vi "Festo.vi"(0 "CloseVi?":bool) -> ()   [LabVIEW 2011]
uses:
  GlobalVariables.vi
panel:
  in  "Valve Mode":bool
  in  "DeviceNet Reset":bool
  in  "DeviceNet HaltScanner":bool
  in  "DeviceNet DisableNetwork":bool
  in  "DeviceNet Fault":bool
  out "DnetPowerDetect":bool
  out "DupNodeFail":bool
  out "CommFailure":bool
  out "Autoverify":bool
  out "DeviceFailure":bool
  out "DisableNetwork":bool
  out "Fault":bool
  out "Run":bool
  out "FB8 Status":bool
  out "FB7 Status":bool
  out "FB6 Status":bool
  out "FB5 Status":bool
  out "FB4 Status":bool
  out "FB3 Status":bool
  out "FB2 Status":bool
  out "FB1 Status":bool
  in  "Close All Valves":bool
  in  "66":bool
  in  "68":bool
  in  "70":bool
  in  "72":bool
  in  "74":bool
  in  "76":bool
  in  "78":bool
  in  "80":bool
  in  "65":bool
  in  "67":bool
  in  "69":bool
  in  "71":bool
  in  "73":bool
  in  "75":bool
  in  "77":bool
  in  "79":bool
  in  "82":bool
  in  "84":bool
  in  "86":bool
  in  "88":bool
  in  "90":bool
  in  "92":bool
  in  "94":bool
  in  "96":bool
  in  "81":bool
  in  "83":bool
  in  "85":bool
  in  "87":bool
  in  "89":bool
  in  "91":bool
  in  "93":bool
  in  "95":bool
  in  "98":bool
  in  "100":bool
  in  "102":bool
  in  "104":bool
  in  "106":bool
  in  "108":bool
  in  "110":bool
  in  "112":bool
  in  "97":bool
  in  "99":bool
  in  "101":bool
  in  "103":bool
  in  "105":bool
  in  "107":bool
  in  "109":bool
  in  "111":bool
  in  "114":bool
  in  "116":bool
  in  "118":bool
  in  "120":bool
  in  "122":bool
  in  "124":bool
  in  "126":bool
  in  "128":bool
  in  "113":bool
  in  "115":bool
  in  "117":bool
  in  "119":bool
  in  "121":bool
  in  "123":bool
  in  "125":bool
  in  "127":bool
  in  "63":bool
  in  "61":bool
  in  "59":bool
  in  "57":bool
  in  "55":bool
  in  "53":bool
  in  "51":bool
  in  "49":bool
  in  "64":bool
  in  "62":bool
  in  "60":bool
  in  "58":bool
  in  "56":bool
  in  "54":bool
  in  "52":bool
  in  "50":bool
  in  "47":bool
  in  "45":bool
  in  "43":bool
  in  "41":bool
  in  "39":bool
  in  "37":bool
  in  "35":bool
  in  "33":bool
  in  "48":bool
  in  "46":bool
  in  "44":bool
  in  "42":bool
  in  "40":bool
  in  "38":bool
  in  "36":bool
  in  "34":bool
  in  "DeviceNet Run":bool
  in  "31":bool
  in  "29":bool
  in  "27":bool
  in  "25":bool
  in  "23":bool
  in  "21":bool
  in  "19":bool
  in  "17":bool
  in  "32":bool
  in  "30":bool
  in  "28":bool
  in  "26":bool
  in  "24":bool
  in  "22":bool
  in  "20":bool
  in  "18":bool
  in  "15":bool
  in  "13":bool
  in  "11":bool
  in  "9":bool
  in  "7":bool
  in  "5":bool
  in  "3":bool
  in  "1":bool
  in  "16":bool
  in  "14":bool
  in  "12":bool
  in  "10":bool
  in  "8":bool
  in  "6":bool
  in  "4":bool
  in  "Close":bool
  in  "2":bool
  # "Festo Block 5"
  # "Festo Block 4"
  # "Festo Block 6"
  # "Festo Block 3"
  # "Festo Block 7"
  # "Festo Block 2"
  # "Festo Block 1"
  # "Festo Block 8"
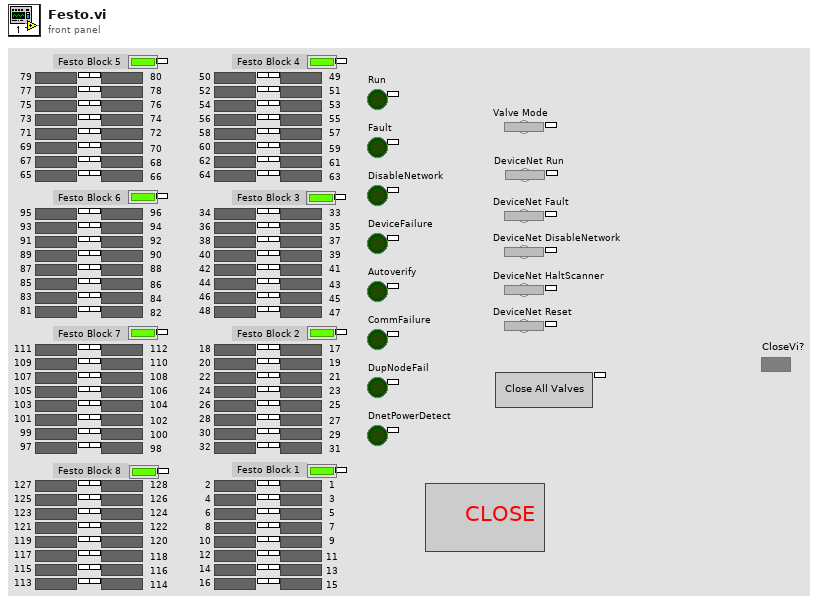
[diagram p1: front panel]
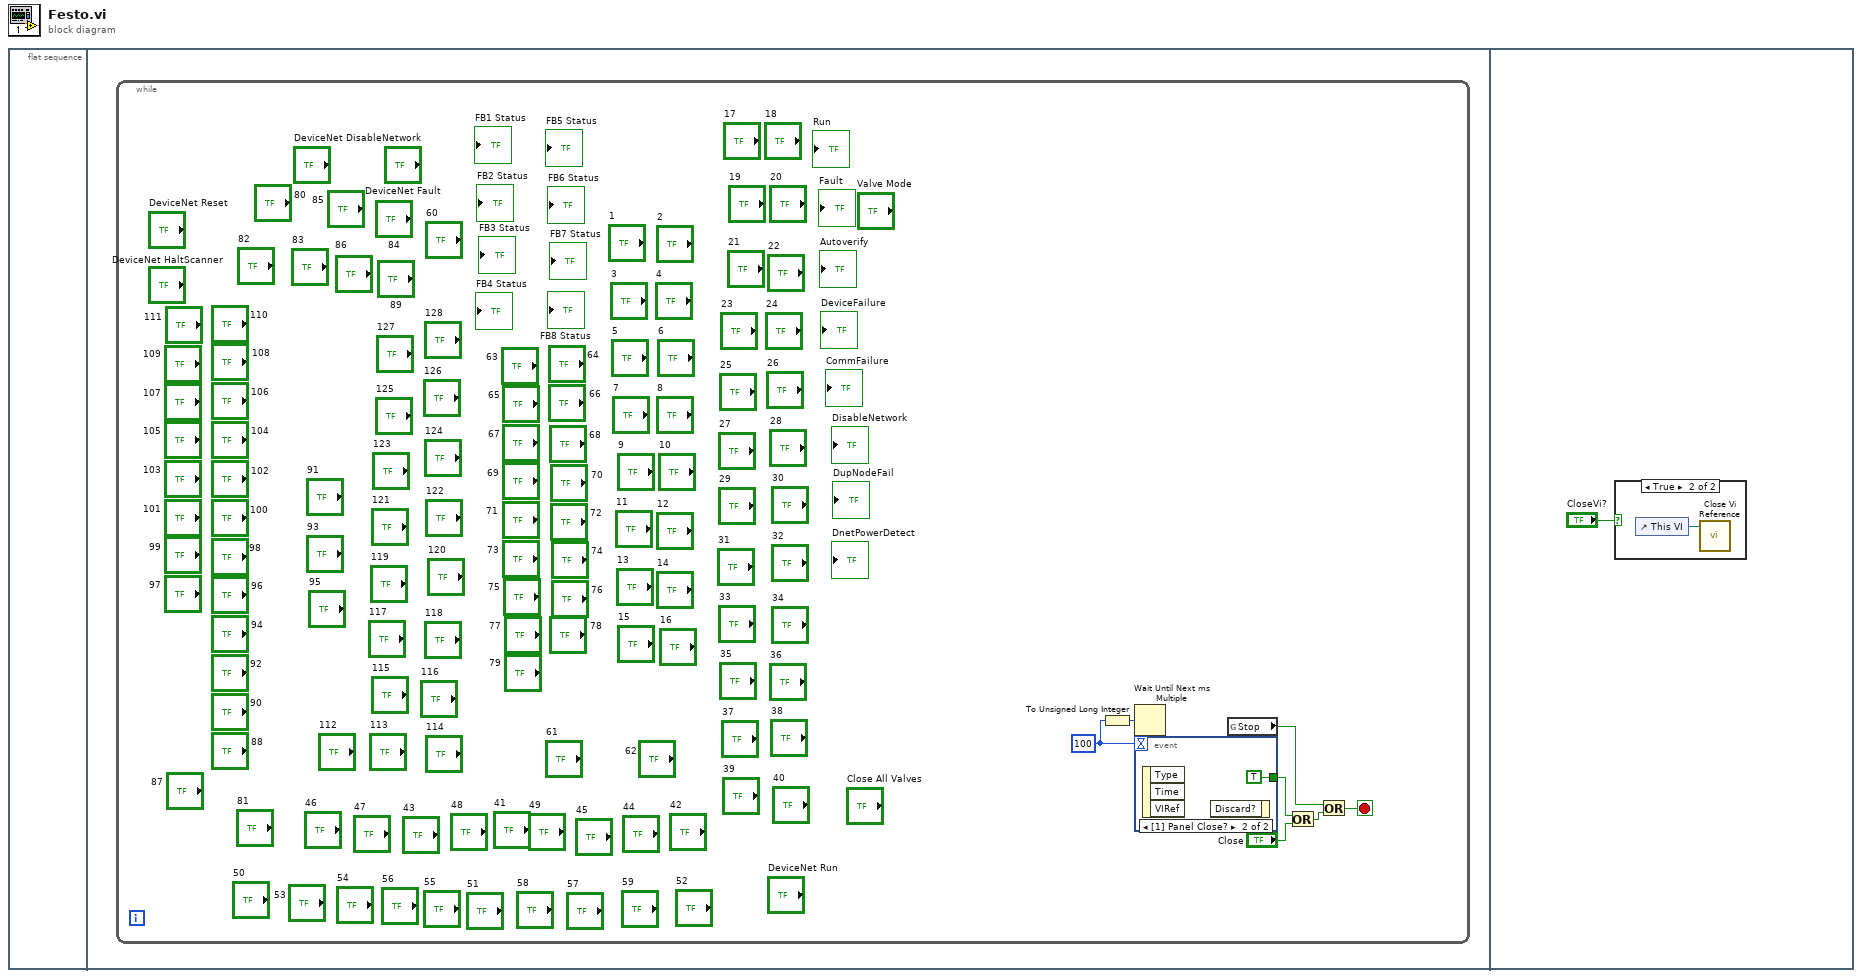
[diagram p0: block diagram]
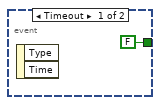
[diagram p2: hidden frame]
diagram:
  n1 = flat-sequence {
    frame #0 {
    }
    frame #1 {
      n2 = while {
        stop <- w3 stop-if-true
        w1 = 100
        n3 = To Unsigned Long Integer(number=w1) -> (unsigned 32bit integer=w2:u32)
        n4 = Wait Until Next ms Multiple(millisecond multiple=w2) -> ()  [unwired: 1 out]
        n5 = event shown="[1] Panel Close?" {
          selector: _ -> [_ _]
          dyn-events: _ -> [_ _]
          timeout: w1 -> [_ _]
          tunnel: [FALSE ("y") TRUE ("y")] -> w4
          event Timeout {
            n6 = event-data() -> ()  [unwired: 1 in, 2 out]
          }
          event Panel Close? {
            n7 = event-data() -> ()  [unwired: 1 in, 3 out]
            n8 = event-data() -> ()  [unwired: 2 in, 1 out]
          }
        }
        n9 = global read "GlobalVariables.vi" "Stop"() -> (w7:bool)
        n10 = Or(x=w4, y="Close") -> (x .or. y?=w6:bool)
        n11 = Or(x=w7, y=w6) -> (x .or. y?=w3:bool)
      }
    }
    frame #2 {
      n12 = case shown="True" "CloseVi?" {
        frame False {
        }
        frame True {
          n13 = control-ref of="This VI"() -> (w11:refnum<vi>)
          n14 = call "Close Vi Reference.vi"("reference"=w11) -> ()  [unwired: 9 in, 2 out]
        }
      }
    }
  }
